vi "Read Expected stripped path.vi"(8 "error in (no error)":errorcluster, 11 "[Test Case] Strip path in":refnum<class "[Test Case] Strip path.lvclass">) -> (0 "error out":errorcluster, 2 "Expected stripped path":string, 3 "[Test Case] Strip path out":refnum<class "[Test Case] Strip path.lvclass">)   [LabVIEW 2016, in "Tests.lvlib" / "[Test Case] Strip path.lvclass"]
uses:
  [Test Case] Strip path.lvclass
  [Test Case] Strip path.lvclass/[Test Case] Strip path.ctl
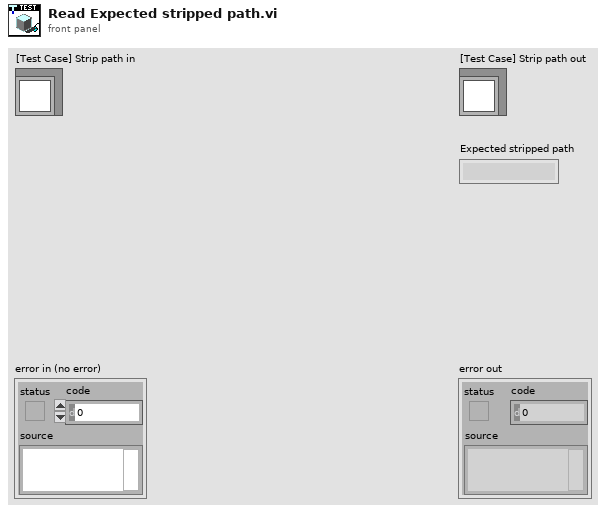
[diagram p1: front panel]
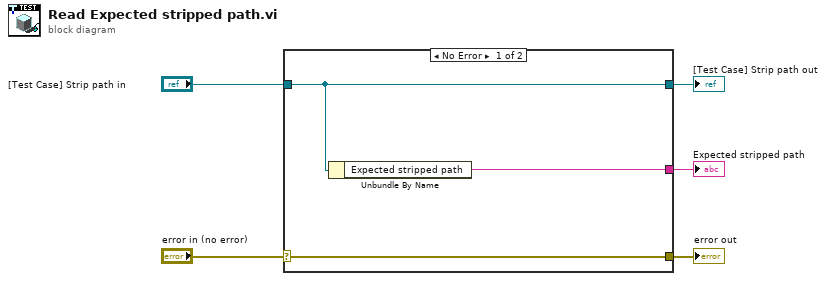
[diagram p0: block diagram]
diagram:
  n1 = case shown="No Error" "error in (no error)" {
    selector: "error in (no error)" -> [w8 w9]
    tunnel: [w8 w9] -> w4
    tunnel: [w7 w10] -> w2
    tunnel: "[Test Case] Strip path in" -> [w7 w10]
    tunnel: [w6 _] -> w1
    frame No Error {
      n2 = Unbundle By Name(w7) -> ("Expected stripped path"=w6:string)
    }
    frame Error {
    }
  }
  "error out" <- w4
  "[Test Case] Strip path out" <- w2
  "Expected stripped path" <- w1
